vi "sv_Compute Frame and Perspective for Octave.vi"(0 "x scale":cluster{"x min":dbl, "x max":dbl} {"x max" format="%.2f"; "x min" format="%.2f"}, 1 "z scale":cluster{"z min":dbl, "z max":dbl} {"z max" format="%.2f"; "z min" format="%.2f"}, 2 "z axis height [%]":dbl format="%.2f", 3 "X maximum":dbl format="%.2f", 4 "Y maximum":dbl format="%.2f") -> (6 "front frame":cluster{dbl[], dbl[]} {"?" format="%.2f"; "?" format="%.2f"}, 7 "back frame":cluster{dbl[], dbl[]} {"?" format="%.2f"; "?" format="%.2f"}, 9 "dY":dbl format="%.2f", 10 "dX":dbl format="%.2f")   [LabVIEW 2017]
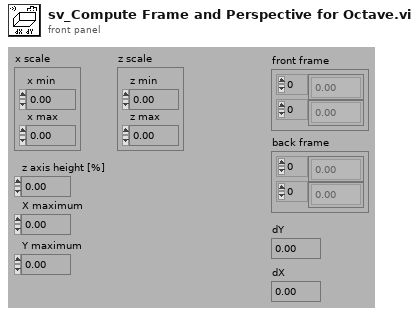
[diagram p1: front panel]
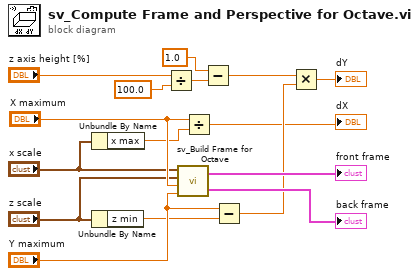
[diagram p0: block diagram]
diagram:
  n1 = Unbundle By Name("x scale") -> ("x max"=w2:dbl)
  n2 = Unbundle By Name("z scale") -> ("z min"=w4:dbl)
  n3 = Divide(x="z axis height [%]", y=100.0) -> (x/y=w9:dbl)
  n4 = call <vilib>:"sv_Build Frame for Octave.vi"("Y maximum"="Y maximum", "X maximum"="X maximum", "z scale"="z scale", "x scale"="x scale") -> ("back frame"=→"back frame":cluster{dbl[], dbl[]}, "front frame"=→"front frame":cluster{dbl[], dbl[]})
  n5 = Divide(x="X maximum", y=w2) -> (x/y=→"dX":dbl)
  n6 = Subtract(x=1.0, y=w9) -> (x-y=w12:dbl)
  n7 = Subtract(x="Y maximum", y=w4) -> (x-y=w13:dbl)
  n8 = Multiply(x=w12, y=w13) -> (x*y=→"dY":dbl)
